vi "_GetBitfieldMask.vi"(10 "size":i32, 11 "offset":i32) -> (3 "mask":u64 format="%.0b")   [LabVIEW 2015, in "Bitfield.lvlib"]
uses:
  Bitfield.lvlib
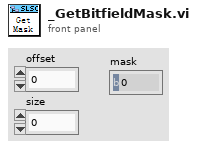
[diagram p1: front panel]
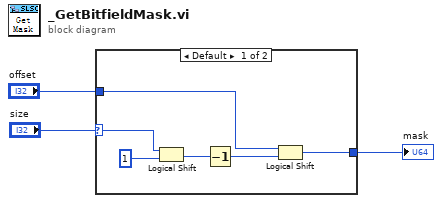
[diagram p0: block diagram]
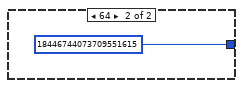
[diagram p2: hidden frame]
diagram:
  n1 = case shown="Default" "size" {
    selector: "size" -> [w8 _]
    tunnel: [w4 u64 18446744073709551615] -> w1
    tunnel: "offset" -> [w5 _]
    frame Default {
      n2 = Logical Shift(y=w8, x=u64 1) -> (x << y=w7:u64)
      n3 = Decrement(x=w7) -> (x-1=w6:u64)
      n4 = Logical Shift(y=w5, x=w6) -> (x << y=w4:u64)
    }
    frame 64 {
    }
  }
  "mask" <- w1
